vi "mod_Calculate AM-SSB impairments.vi"(0 "IF sampling frequency":dbl=2.0, 2 "downconversion filter length":i32=34, 5 "frequency offset (normalized)":dbl, 7 "phase offset (degrees)":dbl, 9 "approx. pilot tone (normalized)":dbl, 11 "error in (no error)":errorcluster) -> (4 "measurements":T1, 15 "error out":errorcluster)   [LabVIEW 2020, in "niAMT.lvlib"]
uses:
  <vilib>/addons/Modulation/niAMT.lvlib
  <vilib>/addons/Modulation/Analog/controls/mod_AM Measurements.ctl
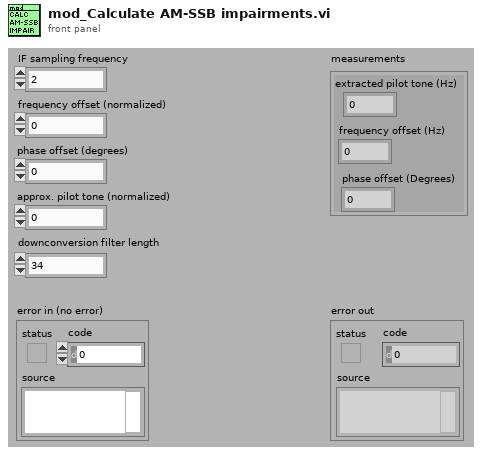
[diagram p1: front panel]
types:
  T1 = typedef "niAMT.lvlib/mod_AM Measurements.ctl" = cluster{"extracted pilot tone (Hz)":dbl, "phase offset (Degrees)":dbl, "frequency offset (Hz)":dbl}
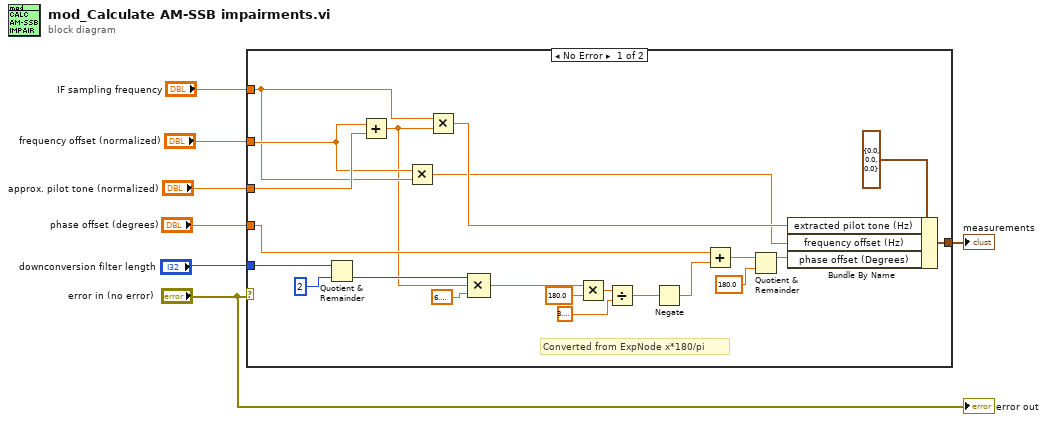
[diagram p0: block diagram]
diagram:
  n1 = case shown="No Error" "error in (no error)" {
    tunnel: "IF sampling frequency" -> [w16 _]
    tunnel: "downconversion filter length" -> [w29 _]
    tunnel: "approx. pilot tone (normalized)" -> [w25 _]
    tunnel: "phase offset (degrees)" -> [w23 _]
    tunnel: "frequency offset (normalized)" -> [w19 _]
    tunnel: [w17 _] -> w2
    frame No Error {
      # "Converted from ExpNode x*180/pi"
      n2 = Quotient & Remainder(x=w29, y=2) -> (floor(x/y)=w27:i32)  [unwired: 1 out]
      n3 = Add(x=w19, y=w25) -> (x+y=w15:dbl)
      n4 = Multiply(x=w19, y=w16) -> (x*y=w18:dbl)
      n5 = Multiply(x=w16, y=w15) -> (x*y=w20:dbl)
      n6 = Compound Arithmetic op=MULTIPLY(w27, w15, 6.283185307179586) -> (w9:dbl)
      n7 = Multiply(x=w9, y=180.0) -> (x*y=w11:dbl)
      n8 = Divide(x=w11, y=3.141592653589793) -> (x/y=w8:dbl)
      n9 = Negate(x=w8) -> (-x=w24:dbl)
      n10 = Add(x=w23, y=w24) -> (x+y=w21:dbl)
      n11 = Quotient & Remainder(x=w21, y=180.0) -> (x-y*floor(x/y)=w14:dbl)  [unwired: 1 out]
      n12 = Bundle By Name(cluster=T1 {"extracted pilot tone (Hz)"=0.0, "phase offset (Degrees)"=0.0, "frequency offset (Hz)"=0.0} ("Measurements"), "extracted pilot tone (Hz)"=w20, "frequency offset (Hz)"=w18, "phase offset (Degrees)"=w14) -> (w17:T1)
    }
    frame Error {
    }
  }
  "measurements" <- w2
  "error out" <- "error in (no error)"
